vi "Turret_Hardware_Globals.vi"() -> ()   [LabVIEW 2019]
panel:
  in  "Turret_Motor":string="Turret_Motor"
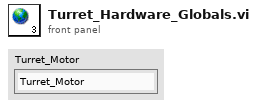
[diagram p1: front panel]
diagram:
